vi "例程44-while和case计数器.vi"() -> ()   [LabVIEW 2016]
panel:
  out "循环次数":u32
  out "点击次数":u32
  in  "停止":bool
  in  "点击":bool
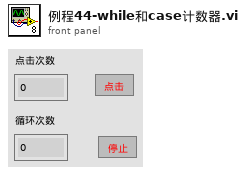
[diagram p1: front panel]
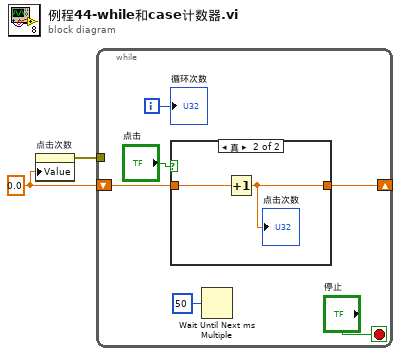
[diagram p0: block diagram]
diagram:
  w2 = 0.0
  n1 = property on="点击次数" class="DigNum (严格)"("Value"=w2) -> (error out=w1:errorcluster)  [unwired: 2 in, 1 out]
  n2 = while {
    shift-right: [w6] -> _
    shift-left: w2 -> [w7]
    tunnel: w1 -> [_]
    i -> [w5]
    stop <- "停止" stop-if-true
    n3 = case shown="真" "点击" {
      tunnel: w7 -> [w9 w11]
      tunnel: [w9 w10] -> w6
      frame False {
      }
      frame True {
        n4 = Increment(x=w11) -> (x+1=w10:dbl)
        "点击次数" <- w10
      }
    }
    n5 = Wait Until Next ms Multiple(millisecond multiple=u32 50 ("毫秒倍数")) -> ()  [unwired: 1 out]
    "循环次数" <- w5
  }
